vi "suma.vi"() -> ()   [LabVIEW 2021]
panel:
  in  "B":dbl
  out "A+B":dbl
  in  "A":dbl
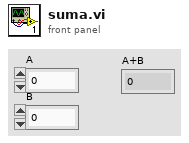
[diagram p1: front panel]
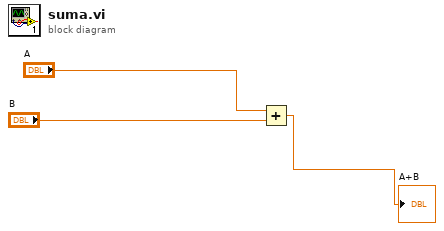
[diagram p0: block diagram]
diagram:
  n1 = Add(x="A", y="B") -> (x+y=→"A+B":dbl)
